vi "NiFPGA Stop FIFO.vi"(8 "error in (no error)":errorcluster, 10 "FIFO":u32, 11 "Session":u32) -> (0 "error out":errorcluster, 3 "Session Out":u32)   [LabVIEW 2010, in "FPGA Interface Wrapper.lvlib"]
doc: "Stops a FIFO."
uses:
  <userlib>/_FPGA Interface Advanced Tools/FPGA Interface Wrapper/FPGA Interface Wrapper.lvlib
  NiFpga.dll
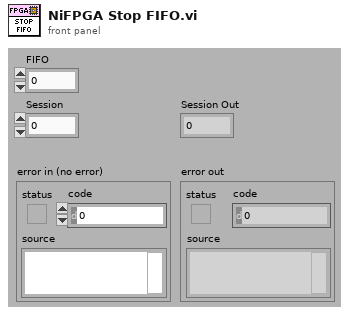
[diagram p1: front panel]
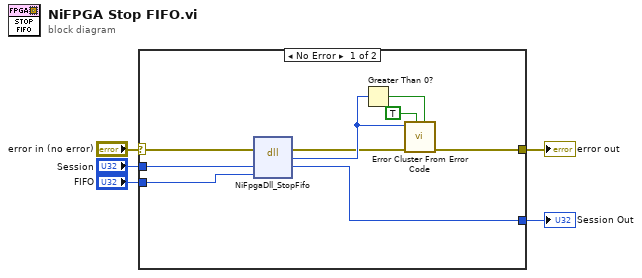
[diagram p0: block diagram]
diagram:
  n1 = case shown="No Error" "error in (no error)" {
    selector: "error in (no error)" -> [w14 w15]
    tunnel: [w6 w15] -> w4
    tunnel: "Session" -> [w13 w16]
    tunnel: [w12 w16] -> w2
    tunnel: "FIFO" -> [w11 _]
    frame No Error {
      n2 = dll-call lib="NiFpga.dll" fn="NiFpgaDll_StopFifo"(error in=w14, "Session"=w13, "FIFO"=w11) -> (error out=w7:errorcluster, "Status"=w8:i32, "Session"=w12:u32)  [unwired: 3 in, 1 out]
      n3 = Greater Than 0?(x=w8) -> (x > 0?=w9:bool)
      n4 = call <vilib>:"Error Cluster From Error Code.vi"("is warning? (False)"=w9, "show call chain? (False)"=TRUE, "error in (no error)"=w7, "error code (0)"=w8) -> ("error out"=w6:errorcluster)  [unwired: 5 in]
    }
    frame Error {
    }
  }
  "error out" <- w4
  "Session Out" <- w2
